vi "Generator Error Strings Global.vi"() -> ()   [LabVIEW 2021]
panel:
  out "5100":string="Internal error. No case found for the control name '%s'."
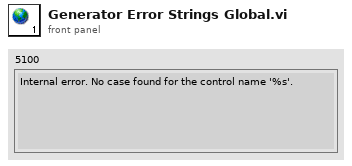
[diagram p1: front panel]
diagram:
